vi "Get Valid Corner Coordinates.vi"(7 "Reference Image":T1(plugin-control), 8 "Error In":errorcluster, 10 "Coordinates":cluster{"X":sgl, "Y":sgl}[](array[cluster])) -> (0 "Error Out":errorcluster, 2 "Corners":cluster{"X":sgl, "Y":sgl}[](array[cluster]))   [LabVIEW 2018]
uses:
  Table Data.vi
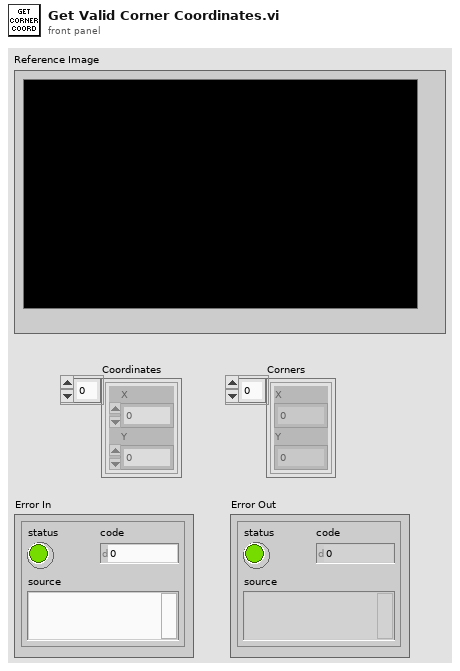
[diagram p1: front panel]
types:
  T1 = typedef "IMAQ Image.ctl" = refnum<image>
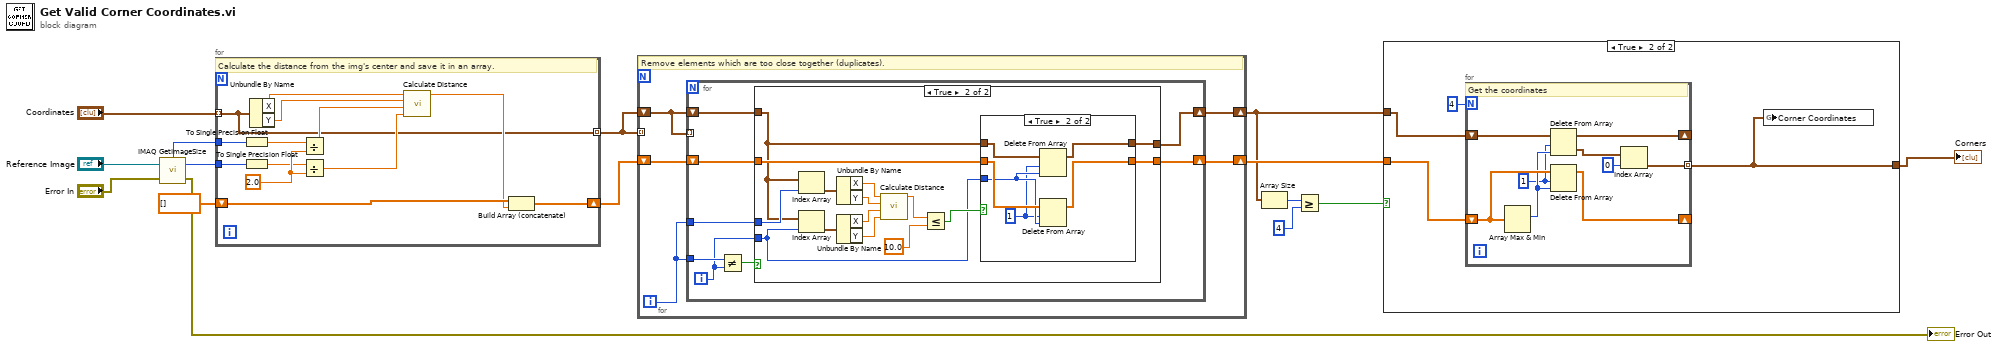
[diagram p0: block diagram]
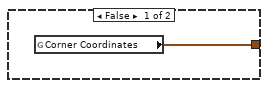
[diagram p2: hidden frame]
diagram:
  n1 = call "IMAQ GetImageSize"("Image"="Reference Image", "error in (no error)"="Error In") -> ("Y Resolution"=w10:i32, "X Resolution"=w9:i32, "error out"=→"Error Out":errorcluster)  [unwired: 2 in]
  n2 = for {
    tunnel: "Coordinates" -> [w20] mode=indexing
    tunnel: w10 -> [w27]
    tunnel: w9 -> [w26]
    shift-right: [w22] -> w14
    shift-left: sgl[] [] -> [w23]
    tunnel: [w20] -> w13 mode=indexing
    w28 = sgl 2.0
    # "Calculate the distance from the img's center and save it in an array."
    n3 = To Single Precision Float(number=w26) -> (single precision float=w19:sgl)
    n4 = To Single Precision Float(number=w27) -> (single precision float=w18:sgl)
    n5 = Unbundle By Name(w20) -> ("X"=w17:sgl, "Y"=w16:sgl)
    n6 = Divide(x=w19, y=w28) -> (x/y=w25:sgl)
    n7 = Divide(x=w18, y=w28) -> (x/y=w24:sgl)
    n8 = call "Calculate Distance.vi"("X1"=w17, "Y1"=w16, "X2"=w25, "Y2"=w24) -> ("Distance"=w21:sgl)  [unwired: 6 in]
    n9 = Build Array (concatenate)(w23, w21) -> (w22:sgl[])
  }
  n10 = for {
    shift-right: [w33] -> w5
    shift-left: w13 -> [w30]
    shift-right: [w31] -> w6
    shift-left: w14 -> [w32]
    tunnel: w13 -> [_] mode=indexing
    i -> [w29]
    # "Remove elements which are too close together (duplicates)."
    n11 = for {
      tunnel: w29 -> [w41]
      shift-right: [w37] -> w33
      shift-left: w30 -> [w38]
      shift-right: [w36] -> w31
      shift-left: w32 -> [w39]
      tunnel: w30 -> [_] mode=indexing
      tunnel: w29 -> [w34]
      i -> [w35]
      n12 = Not Equal?(x=w41, y=w35) -> (x != y?=w40:bool)
      n13 = case shown="True" w40 {
        tunnel: w39 -> [w42 w48]
        tunnel: w38 -> [w43 w46]
        tunnel: [w43 w45] -> w37
        tunnel: [w42 w47] -> w36
        tunnel: w35 -> [_ w44]
        tunnel: w34 -> [_ w58]
        frame False {
        }
        frame True {
          n14 = Index Array(array=w46, index=w58) -> (element=w57:cluster{"X":sgl, "Y":sgl})
          n15 = Index Array(array=w46, index=w44) -> (element=w56:cluster{"X":sgl, "Y":sgl})
          n16 = Unbundle By Name(w57) -> ("X"=w55:sgl, "Y"=w54:sgl)
          n17 = Unbundle By Name(w56) -> ("X"=w53:sgl, "Y"=w52:sgl)
          n18 = call "Calculate Distance.vi"("X1"=w55, "Y1"=w54, "X2"=w53, "Y2"=w52) -> ("Distance"=w51:sgl)  [unwired: 6 in]
          n19 = Less Or Equal?(x=w51, y=sgl 10.0) -> (x <= y?=w49:bool)
          n20 = case shown="True" w49 {
            tunnel: w48 -> [w60 w65]
            tunnel: [w60 w61] -> w47
            tunnel: w46 -> [w59 w66]
            tunnel: [w59 w62] -> w45
            tunnel: w44 -> [_ w64]
            frame False {
            }
            frame True {
              w63 = 1 ("length")
              n21 = Delete From Array(array=w66, length=w63, index=w64) -> (array with subset deleted=w62:cluster{"X":sgl, "Y":sgl}[])  [unwired: 1 out]
              n22 = Delete From Array(array=w65, length=w63, index=w64) -> (array with subset deleted=w61:sgl[])  [unwired: 1 out]
            }
          }
        }
      }
    }
  }
  n23 = Array Size(array=w5) -> (size(s)=w12:i32)
  n24 = Greater Or Equal?(x=w12, y=4) -> (x >= y?=w7:bool)
  n25 = case shown="True" w7 {
    tunnel: w6 -> [_ w70]
    tunnel: w5 -> [_ w69]
    tunnel: [w67 w68] -> w2
    frame False {
      n26 = global read "Table Data.vi" "Corner Coordinates"() -> (w67:cluster{"X":sgl, "Y":sgl}[])
    }
    frame True {
      n27 = for {
        N: 4 -> [_]
        shift-right: [w79] -> _
        shift-left: w70 -> [w80]
        tunnel: [w72] -> w68 mode=indexing
        shift-right: [w75] -> _
        shift-left: w69 -> [w78]
        w76 = 1 ("length")
        # "Get the coordinates"
        n28 = Array Max & Min(array=w80) -> (max index (indices)=w77:i32)  [unwired: 3 out]
        n29 = Delete From Array(array=w78, length=w76, index=w77) -> (deleted portion=w74:cluster{"X":sgl, "Y":sgl}[], array with subset deleted=w75:cluster{"X":sgl, "Y":sgl}[])
        n30 = Delete From Array(array=w80, length=w76, index=w77) -> (array with subset deleted=w79:sgl[])  [unwired: 1 out]
        n31 = Index Array(array=w74, index=0) -> (element=w72:cluster{"X":sgl, "Y":sgl})
      }
      n32 = global write "Table Data.vi" "Corner Coordinates"(w68) -> ()
    }
  }
  "Corners" <- w2
